vi "Rechnungsdaten.vi"() -> ()   [LabVIEW 2023]
panel:
  in  "PLZ":dbl
  in  "Ort":string
  in  "Straße":string
  in  "Firmenname":string
  out "Firma":bool
  in  "Blank Button 3":bool
  in  "Blank Button 2":bool
  in  "Blank Button":bool
  in  "Stop Button":bool
  in  "Nachname":string
  in  "Vorname":string
  out "error out":errorcluster
  in  "error in (no error)":errorcluster
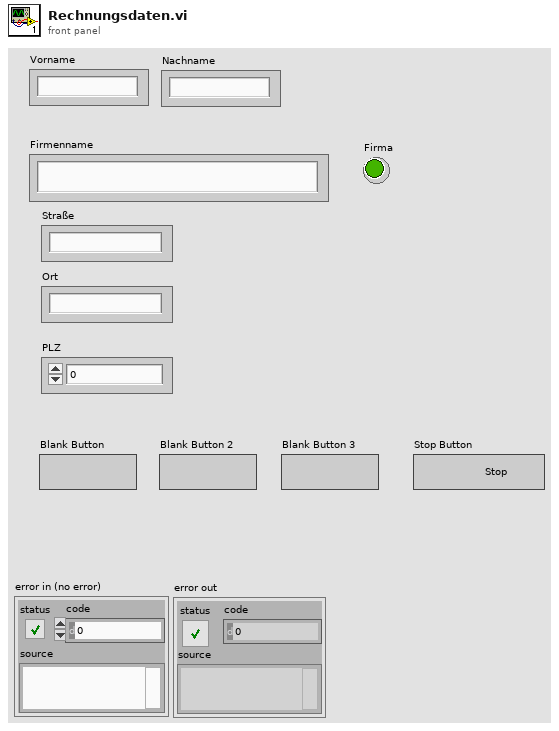
[diagram p1: front panel]
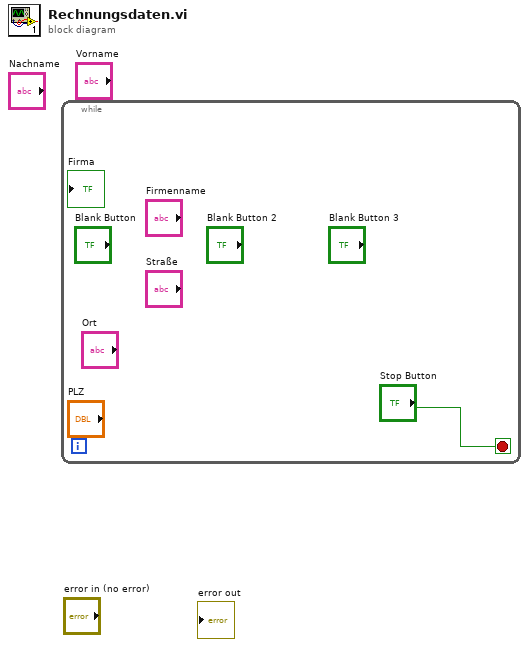
[diagram p0: block diagram]
diagram:
  n1 = while {
    stop <- "Stop Button" stop-if-true
  }
